vi "Result_Test.vi"(8 "error in (no error)":errorcluster caption="entrée d'erreur (pas d'erreur)", 11 "Generate_SN en entrée":refnum<class "Generate_SN.lvclass">) -> (0 "error out":errorcluster caption="sortie d'erreur", 3 "Generate_SN en sortie":refnum<class "Generate_SN.lvclass">)   [LabVIEW 2020, in "Library Test.lvlib" / "Generate_SN.lvclass"]
uses:
  Generate_SN.lvclass
  C:/Users/ngarcin/OneDrive - Altyor/Standard TB/Suite TB45/Class/Test/Test (Default)/Test (Default).lvclass
  Commun VI/TypeDef/Variable Printable.ctl
  Test_Without_Instr/Test_Without_Inst.lvclass
  Commun VI/Library Commun.lvlib
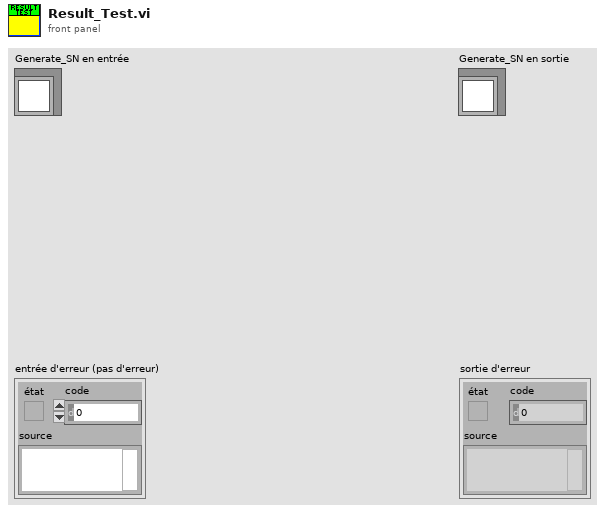
[diagram p1: front panel]
types:
  T1 = enum16{"Get Variable", "Get All Variables", "Set Variable", "Delete Variable", "Delete All Variable"}
  T2 = typedef "Variable Printable.ctl" = string
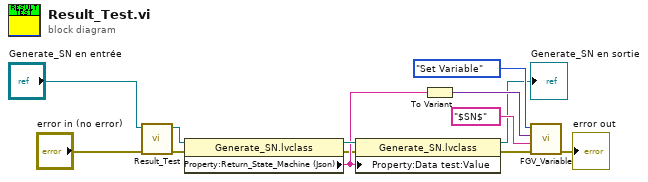
[diagram p0: block diagram]
diagram:
  n1 = call-parent "Result_Test.vi"("error in (no error)"="error in (no error)", "Test_Without_Inst en entrée"="Generate_SN en entrée") -> ("error out"=w6:errorcluster, "Test_Without_Inst en sortie"=w7:refnum<class "Generate_SN.lvclass">)  [unwired: 8 in]
  n2 = property class="Generate_SN.lvclass"(reference=w7, error in=w6) -> (reference out=w5:refnum<class "Generate_SN.lvclass">, error out=w3:errorcluster, "Property:Return_State_Machine (Json)"=w4:string)
  n3 = property class="Generate_SN.lvclass"(reference=w5, error in=w3, "Property:Data test:Value"=w4) -> (reference out=→"Generate_SN en sortie":refnum<class "Generate_SN.lvclass">, error out=w2:errorcluster)
  n4 = To Variant(anything=w4) -> (Variant=w9:variant)
  n5 = call "FGV_Variable.vi"("error in (no error)"=w2, "Variable"=T2 "$SN$" ("Variable Printable"), "Data In"=w9, "Function"=T1."Set Variable") -> ("error out"=→"error out":errorcluster)  [unwired: 5 in, 2 out]
